vi "TestControlVi.vi"() -> ()   [LabVIEW 2018]
panel:
  out "file path":path=path "E:/Materials Testing/2018-05-15/Run13Sensors.tdms"
  in  "File Information":T1={"Project"=enum."H2TC", "SubFolder"="VAPORTUBE\\Temp Dependence", "Filename (Meas. Description)"="Power_80C", "Measurement number"=0}
  out "tdms error":errorcluster
  out "tdms file":refnum<k34>
  out "output cluster":cluster{"Sine with Uniform Noise":dynamicdata}
  out "Sine with Uniform Noise":dbl=0.05394995810837566
  in  "stop":bool
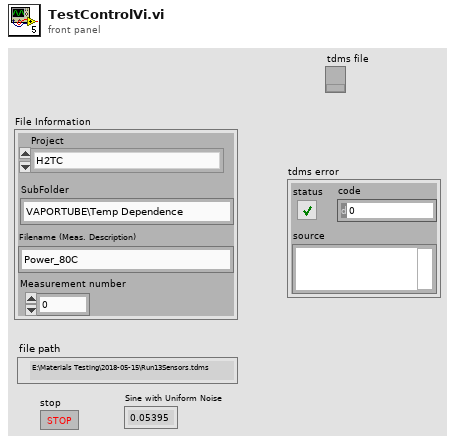
[diagram p1: front panel]
types:
  T1 = cluster{"Project":enum16{"H2TC", "VAPOR1"}, "SubFolder":string, "Filename (Meas. Description)":string, "Measurement number":i32}
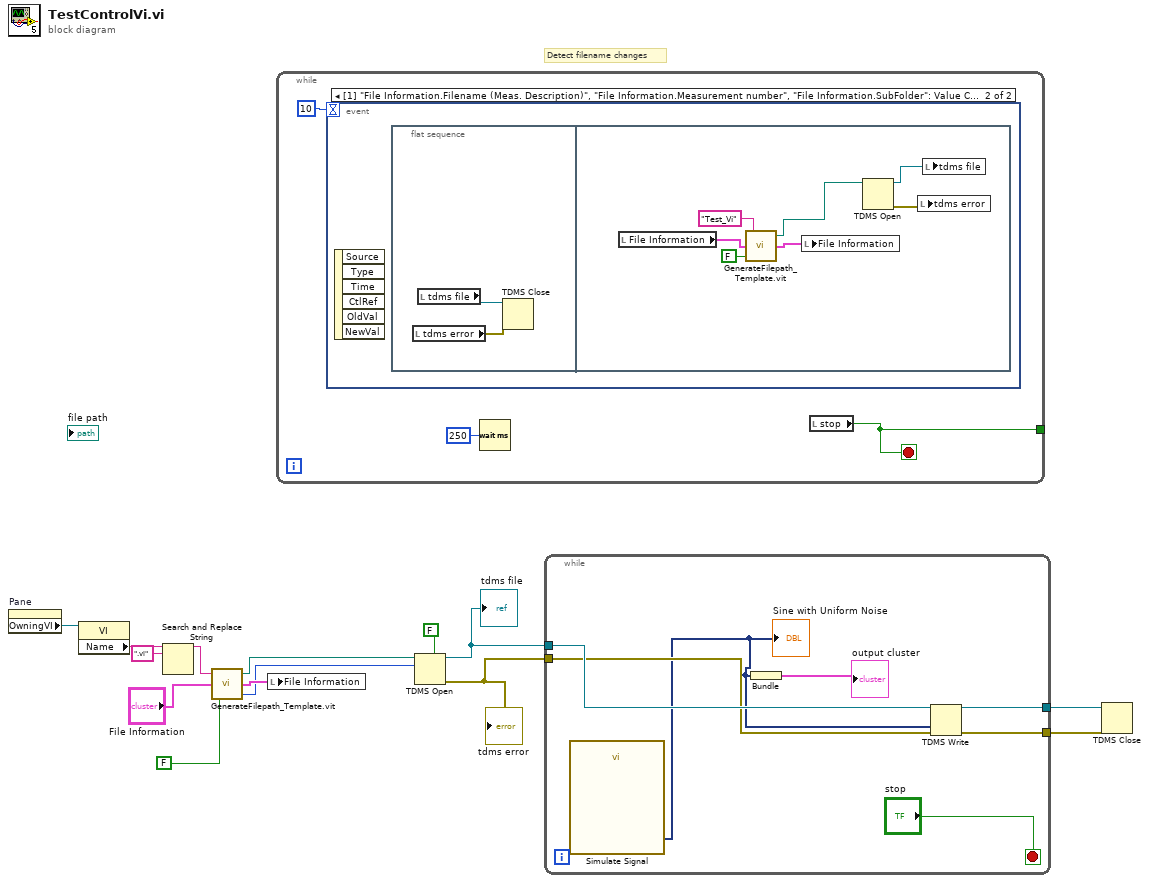
[diagram p0: block diagram]
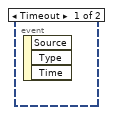
[diagram p2: hidden frame]
diagram:
  # "Detect filename changes"
  n1 = property on="Pane" class="Pane"() -> ("OwningVI"=w9:refnum<vi>)  [unwired: 2 in, 2 out]
  n2 = property class="VI"(reference=w9) -> ("Name"=w8:string)  [unwired: 1 in, 2 out]
  n3 = Search and Replace String(input string=w8, search string=".vi") -> (result string=w6:string)  [unwired: 6 in, 3 out]
  n4 = call "GenerateFilepath_Template.vit"("Check for file?"=FALSE, "File Information"="File Information", "Instrument"=w6) -> ("File Action"=w10:i32, "File Information Out"=w12:T1, "File Path Out"=w11:path)
  n5 = local write "File Information"(w12) -> ()
  n6 = while {
    tunnel: [w15] -> _
    stop <- w15 stop-if-true
    n7 = event shown="[1] \"File Information.Filename (Meas. Description)\", \"File Information.Measurement number\", \"File Information.SubFolder\": Value Change" {
      selector: _ -> [_ _]
      dyn-events: _ -> [_ _]
      timeout: 10 -> [_ _]
      event Timeout {
        n8 = event-data() -> ()  [unwired: 1 in, 3 out]
      }
      event "File Information.Filename (Meas. Description)", "File Information.Measurement number", "File Information.SubFolder": Value Change {
        n9 = event-data() -> ()  [unwired: 1 in, 6 out]
        n10 = flat-sequence {
          frame #0 {
            n11 = local read "tdms error"() -> (w19:errorcluster)
            n12 = local read "tdms file"() -> (w18:refnum<k34>)
            n13 = TDMS Close(8:w19, 11:w18) -> ()  [unwired: 2 out]
          }
          frame #1 {
            n14 = local read "File Information"() -> (w24:T1)
            n15 = call "GenerateFilepath_Template.vit"("Check for file?"=FALSE, "File Information"=w24, "Instrument"="Test_Vi") -> ("File Information Out"=w26:T1, "File Path Out"=w23:path)  [unwired: 1 out]
            n16 = local write "File Information"(w26) -> ()
            n17 = TDMS Open(11:w23) -> (0:w21:errorcluster, 3:w22:refnum<k34>)  [unwired: 6 in]
            n18 = local write "tdms error"(w21) -> ()
            n19 = local write "tdms file"(w22) -> ()
          }
        }
      }
    }
    n20 = Wait (ms)(milliseconds to wait=u32 250) -> ()  [unwired: 1 out]
    n21 = local read "stop"() -> (w15:bool)
  }
  n22 = TDMS Open(5:FALSE ("create index file? (T)"), 10:w10, 11:w11) -> (0:w3:errorcluster, 3:w4:refnum<k34>)  [unwired: 4 in]
  "tdms file" <- w4
  "tdms error" <- w3
  n23 = while {
    tunnel: w4 -> [w31]
    tunnel: w3 -> [w30]
    tunnel: [w28] -> w1
    tunnel: [w27] -> w2
    stop <- "stop" stop-if-true
    n24 = call "Simulate Signal"() -> ("Sine with Uniform Noise"=w29:dynamicdata)  [unwired: 14 in, 1 out]
    "Sine with Uniform Noise" <- w29
    n25 = Bundle("Sine with Uniform Noise"=w29) -> (→"output cluster":cluster{"Sine with Uniform Noise":dynamicdata})  [unwired: 1 in]
    n26 = TDMS Write(0:w31, 9:w29, 11:w30) -> (4:w28:refnum<k34>, 15:w27:errorcluster)  [unwired: 3 in, 2 out]
  }
  n27 = TDMS Close(8:w2, 11:w1) -> ()  [unwired: 2 out]
